vi "UT_001_TOML to LV.vi"() -> ()   [LabVIEW 2017]
uses:
  b63e0b88-7ba7-4dee-a43e-fc5dcdf3e80e.vi
  7dc6aa98-3bd4-4305-a38f-b45c177b78e8.vi
  c5341fb9-8734-4d16-865c-83784ba59dbe.vi
  9b204452-4378-4217-8ce8-edfe2d471006.vi
  04455632-4ea7-4004-ad0e-dcc5f65a6605.vi
  88135e47-21b0-4fd1-85e0-e7ee9c587d2f.vi
  lib/TOML to LabVIEW.vi
  <vilib>/addons/_JKI Toolkits/Caraya/classes/Assert/Assert Not Error.vi
  <vilib>/addons/_JKI Toolkits/Caraya/classes/Assert/Assert True.vi
  <vilib>/addons/_JKI Toolkits/Caraya/classes/Assert/Assert Error.vi
  <vilib>/addons/_JKI Toolkits/Caraya/classes/Assert/Assert Equal Value_Variant.vi
  <vilib>/addons/_JKI Toolkits/Caraya/classes/Test/Test.lvclass
  <vilib>/addons/_JKI Toolkits/Caraya/classes/Assert/Assert.lvclass
  lib/TOML.lvlib
panel:
  out "error out":errorcluster
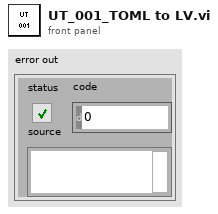
[diagram p1: front panel]
types:
  T1 = cluster{"error":cluster{"sttus":bool, "code":i32, "source":string}}
  T2 = typedef "TOML.lvlib/TOML Value.ctl" = cluster{"type":enum16{"Table", "Array", "String", "Integer", "Float", "Boolean", "Offset Date-Time", "Local Date-Time", "Local Date", "Local Time", "Path"}, "value":variant}
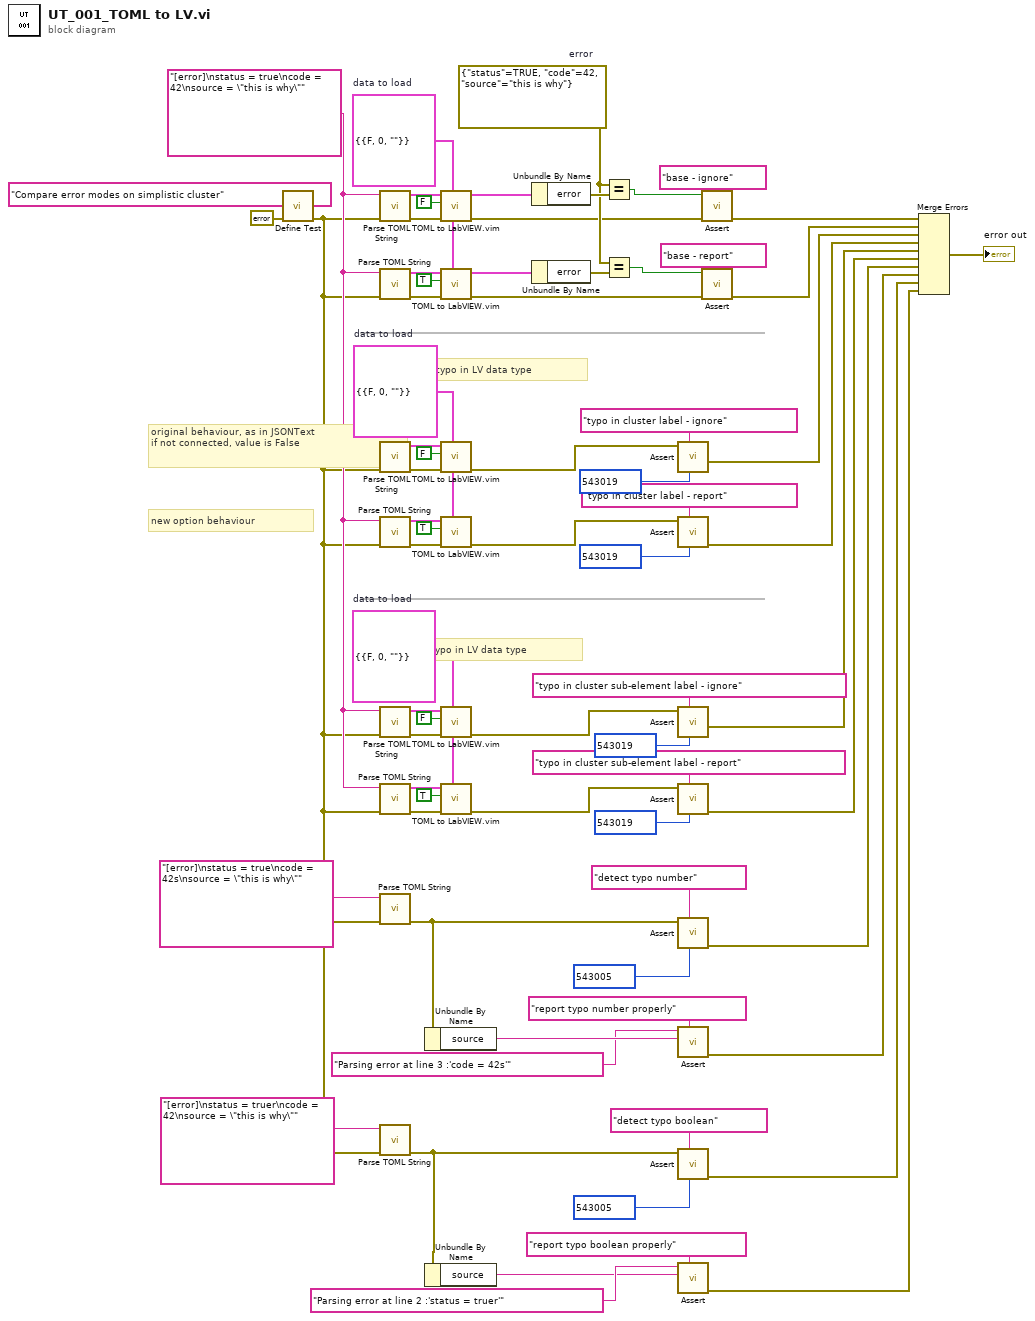
[diagram p0: block diagram]
diagram:
  w33 = T1 {"error"={"sttus"=FALSE, "code"=0, "source"=""}}  # data to load
  w25 = cluster{"errr":errorcluster} {"errr"={"status"=FALSE, "code"=0, "source"=""}}  # data to load
  w44 = cluster{"error":errorcluster} {"error"={"status"=FALSE, "code"=0, "source"=""}}  # data to load
  w57 = errorcluster {"status"=TRUE, "code"=42, "source"="this is why"}  # error
  w51 = "[error]\nstatus = true\ncode = 42\nsource = \"this is why\"" ("String")
  # "new option behaviour"
  # "original behaviour, as in JSONText\nif not connected, value is False"
  # "typo in LV data type"
  # "typo in LV data type"
  n1 = call <vilib>:"Define Test.vi"("error in (no error)"=errorcluster {"status"=FALSE, "code"=0, "source"=""}, "Label (VI Title)"="Compare error modes on simplistic cluster") -> ("error out"=w13:errorcluster)  [unwired: 9 in]
  n2 = call "Parse TOML String.vi"("error in (no error)"=w13, "String"=w51) -> ("error out"=w47:errorcluster, "Value"=w48:T2)  [unwired: 8 in]
  n3 = call "Parse TOML String.vi"("error in (no error)"=w13, "String"=w51) -> ("error out"=w42:errorcluster, "Value"=w45:T2)  [unwired: 8 in]
  n4 = call "Parse TOML String.vi"("error in (no error)"=w13, "String"=w51) -> ("error out"=w23:errorcluster, "Value"=w21:T2)  [unwired: 8 in]
  n5 = call "Parse TOML String.vi"("error in (no error)"=w13, "String"=w51) -> ("error out"=w28:errorcluster, "Value"=w24:T2)  [unwired: 8 in]
  n6 = call "Parse TOML String.vi"("error in (no error)"=w13, "String"=w51) -> ("error out"=w35:errorcluster, "Value"=w37:T2)  [unwired: 8 in]
  n7 = call "Parse TOML String.vi"("error in (no error)"=w13, "String"=w51) -> ("error out"=w30:errorcluster, "Value"=w32:T2)  [unwired: 8 in]
  n8 = call "Parse TOML String.vi"("error in (no error)"=w13, "String"="[error]\nstatus = true\ncode = 42s\nsource = \"this is why\"") -> ("error out"=w11:errorcluster)  [unwired: 8 in, 1 out]
  n9 = call "Parse TOML String.vi"("error in (no error)"=w13, "String"="[error]\nstatus = truer\ncode = 42\nsource = \"this is why\"") -> ("error out"=w2:errorcluster)  [unwired: 8 in, 1 out]
  n10 = Unbundle By Name(w11) -> ("source"=w10:string)
  n11 = Unbundle By Name(w2) -> ("source"=w3:string)
  n12 = call "TOML to LabVIEW.vim"("datatype"=w44, "error in (no error)"=w47, "Error if missing element"=FALSE, "Value"=w48) -> ("error out"=w41:errorcluster, "LV Data"=w46:cluster{"error":errorcluster})  [unwired: 5 in, 1 out]
  n13 = call "TOML to LabVIEW.vim"("datatype"=w44, "error in (no error)"=w42, "Error if missing element"=TRUE, "Value"=w45) -> ("error out"=w40:errorcluster, "LV Data"=w39:cluster{"error":errorcluster})  [unwired: 5 in, 1 out]
  n14 = call "TOML to LabVIEW.vim"("error in (no error)"=w23, "Error if missing element"=FALSE, "Value"=w21) -> ("error out"=w22:errorcluster)  [unwired: 6 in, 2 out]
  n15 = call "TOML to LabVIEW.vim"("datatype"=w25, "error in (no error)"=w28, "Error if missing element"=TRUE, "Value"=w24) -> ("error out"=w26:errorcluster)  [unwired: 5 in, 2 out]
  n16 = call "TOML to LabVIEW.vim"("datatype"=w33, "error in (no error)"=w35, "Error if missing element"=FALSE, "Value"=w37) -> ("error out"=w34:errorcluster)  [unwired: 5 in, 2 out]
  n17 = call "TOML to LabVIEW.vim"("datatype"=w33, "error in (no error)"=w30, "Error if missing element"=TRUE, "Value"=w32) -> ("error out"=w29:errorcluster)  [unwired: 5 in, 2 out]
  n18 = Unbundle By Name(w46) -> ("error"=w67:errorcluster)
  n19 = Unbundle By Name(w39) -> ("error"=w60:errorcluster)
  n20 = Equal?(x=w57, y=w67) -> (x = y?=w69:bool)
  n21 = Equal?(x=w57, y=w60) -> (x = y?=w59:bool)
  n22 = call-poly <vilib>:"Assert.vi"("error code (1)"=543019, "Label"="typo in cluster label - ignore" ("Label (VI Title)"), "Not Error?"=w22) -> ("error out"=w65:errorcluster)  [unwired: 8 in]
  n23 = call-poly <vilib>:"Assert.vi"("error code (1)"=543019, "Label"="typo in cluster label - report" ("Label (VI Title)"), "Error?"=w26) -> ("error out"=w49:errorcluster)  [unwired: 8 in]
  n24 = call-poly <vilib>:"Assert.vi"("error code (1)"=543019, "Label"="typo in cluster sub-element label - ignore" ("Label (VI Title)"), "Not Error?"=w34) -> ("error out"=w63:errorcluster)  [unwired: 8 in]
  n25 = call-poly <vilib>:"Assert.vi"("error code (1)"=543019, "Label"="typo in cluster sub-element label - report" ("Label (VI Title)"), "Error?"=w29) -> ("error out"=w50:errorcluster)  [unwired: 8 in]
  n26 = call-poly <vilib>:"Assert.vi"("error code (1)"=543005, "Label"="detect typo number" ("Label (VI Title)"), "Error?"=w11) -> ("error out"=w12:errorcluster)  [unwired: 8 in]
  n27 = call-poly <vilib>:"Assert.vi"("Label"="report typo number properly" ("Label (VI Title)"), "Y"=w10, "X"="Parsing error at line 3 :'code = 42s'" ("Label (VI Title)")) -> ("error out"=w8:errorcluster)  [unwired: 8 in]
  n28 = call-poly <vilib>:"Assert.vi"("error code (1)"=543005, "Label"="detect typo boolean" ("Label (VI Title)"), "Error?"=w2) -> ("error out"=w9:errorcluster)  [unwired: 8 in]
  n29 = call-poly <vilib>:"Assert.vi"("Label"="report typo boolean properly" ("Label (VI Title)"), "Y"=w3, "X"="Parsing error at line 2 :'status = truer'" ("Label (VI Title)")) -> ("error out"=w1:errorcluster)  [unwired: 8 in]
  n30 = call-poly <vilib>:"Assert.vi"("Label"="base - ignore" ("Label (VI Title)"), "error in (no error)"=w41, "True?"=w69) -> ("error out"=w72:errorcluster)  [unwired: 8 in]
  n31 = call-poly <vilib>:"Assert.vi"("Label"="base - report" ("Label (VI Title)"), "error in (no error)"=w40, "True?"=w59) -> ("error out"=w56:errorcluster)  [unwired: 8 in]
  n32 = Merge Errors(w72, w56, w65, w49, w63, w50, w12, w8, w9, w1) -> (→"error out":errorcluster)
